vi "Read Buffer Size.vi"(11 "Network Stream in":refnum<class "Network Stream.lvclass">) -> (2 "Buffer Size":i32=4096)   [LabVIEW 2020, in "Network Stream.lvclass"]
doc: "This VI returns the buffer size specified for this endpoint of the network stream."
uses:
  Network Stream.lvclass
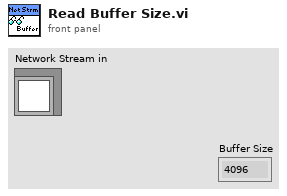
[diagram p1: front panel]
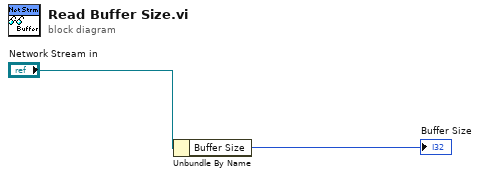
[diagram p0: block diagram]
diagram:
  n1 = Unbundle By Name("Network Stream in") -> ("Buffer Size"=→"Buffer Size":i32)
